vi "tcsOfc_logEvent_loopTimeOutOfRange.vi"(8 "error in (no error)":errorcluster, 11 "logevent_loopTimeOutOfRange_Ctl":T1) -> (0 "error out":errorcluster, 2 "function return":i32, 3 "logevent_loopTimeOutOfRange_Ctl out":T1)   [LabVIEW 2016, in "SALLV_tcsOfc.lvlib"]
doc: "int tcsOfc_shm_logEvent_loopTimeOutOfRangeLV(tcsOfc_logevent_loopTimeOutOfRangeLV *logevent_loopTimeOutOfRange_Ctl );"
uses:
  SALLV_tcsOfc.lvlib
  DataTypes/logevent_loopTimeOutOfRange.ctl
  SALLV_tcsOfc.so
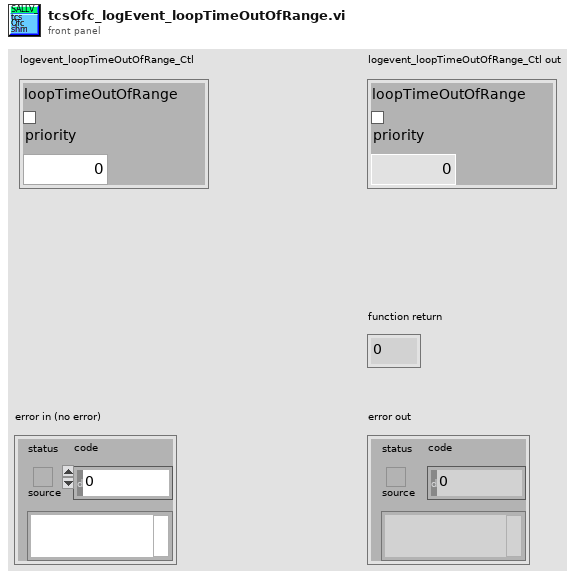
[diagram p1: front panel]
types:
  T1 = typedef "SALLV_tcsOfc.lvlib/logevent_loopTimeOutOfRange.ctl" = cluster{"loopTimeOutOfRange":bool, "priority":i32}
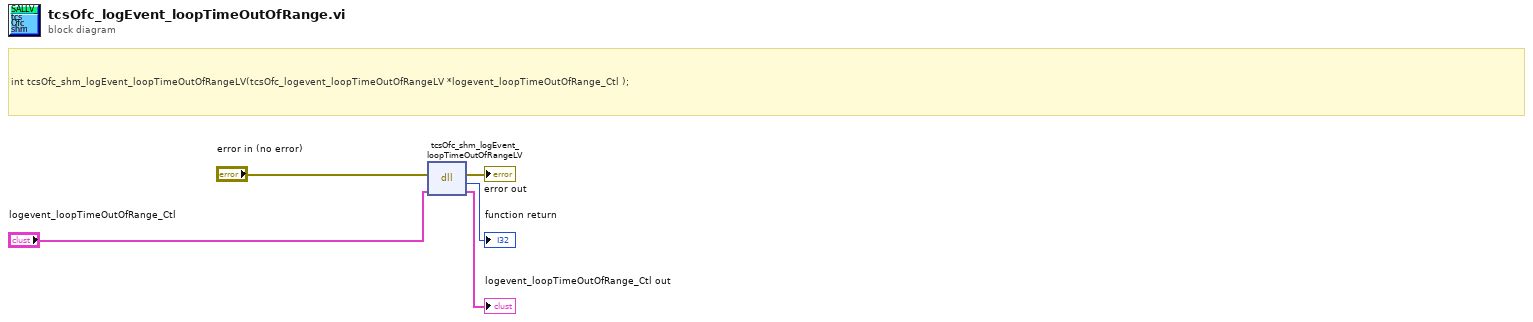
[diagram p0: block diagram]
diagram:
  # "int tcsOfc_shm_logEvent_loopTimeOutOfRangeLV(tcsOfc_logevent_loopTimeOutOfRangeLV *logevent_loopTimeOutOfRange_Ctl );"
  n1 = dll-call lib="home/ttsai/Documents/salAPI/SALLV_tcsOfc/SALLV_tcsOfc.*" fn="tcsOfc_shm_logEvent_loopTimeOutOfRangeLV"(error in="error in (no error)", "logevent_loopTimeOutOfRange_Ctl"="logevent_loopTimeOutOfRange_Ctl") -> (error out=→"error out":errorcluster, →"function return":i32, "logevent_loopTimeOutOfRange_Ctl"=→"logevent_loopTimeOutOfRange_Ctl out":T1)  [unwired: 2 in, 1 out]
